vi "Read applicationHandler.vi"(11 "ComponentData in":refnum<class "ComponentData.lvclass">) -> (2 "ApplicationHandler.lvclass":refnum<class "ApplicationHandler.lvclass">, 3 "ComponentData out":refnum<class "ComponentData.lvclass">)   [LabVIEW 2013, in "ComponentData.lvlib" / "ComponentData.lvclass"]
uses:
  <userlib>/Common/Component/Application/RT/ComponentData/ComponentData/ComponentData.lvclass
  <userlib>/Common/Component/Application/RT/ComponentData/ApplicationHandler/ApplicationHandler.lvclass
  <userlib>/Common/Component/Application/RT/ComponentData/ComponentData/ComponentData.lvclass/ComponentData.ctl
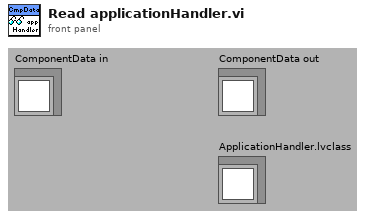
[diagram p1: front panel]
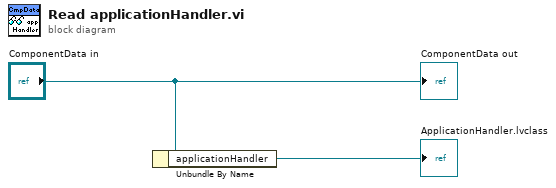
[diagram p0: block diagram]
diagram:
  n1 = Unbundle By Name("ComponentData in") -> ("applicationHandler"=→"ApplicationHandler.lvclass":refnum<class "ApplicationHandler.lvclass">)
  "ComponentData out" <- "ComponentData in"
